vi "SmartSEM Remote API FIB VI slope.vi"(8 "error in":errorcluster, 11 "ActiveX Container":refnum<k7>(container)) -> (0 "error out":errorcluster, 2 "V/I slope":sgl format="%.1g", 3 "reference out":refnum<k7>)   [LabVIEW 2018]
panel:
  in  "Cancel":bool
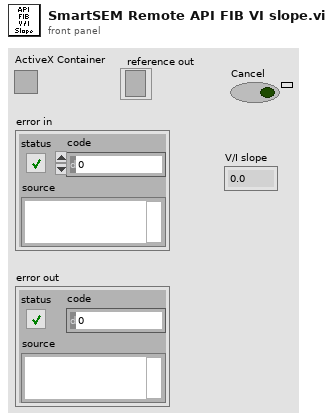
[diagram p1: front panel]
types:
  T1 = cluster{"Filament (A)":sgl, "Accelerator Target (V)":sgl, "Accelerator Actual (V)":sgl, "Extrator Target (V)":sgl, "Extrator Actual (V)":sgl, "Emission Target (uA)":sgl, "Emission Actual (uA)":sgl, "Suppressor (V)":sgl, "Faraday I (nA)":sgl, "Lens1 Target (V)":sgl, "Lens1 Actual (V)":sgl, "Lens2 Target (V)":sgl, "Lens2 Actual (V)":sgl, "Gun Vac (Torr)":sgl, "Column Vac (Torr)":sgl, "Tip Lifetime (uAhr)":sgl}
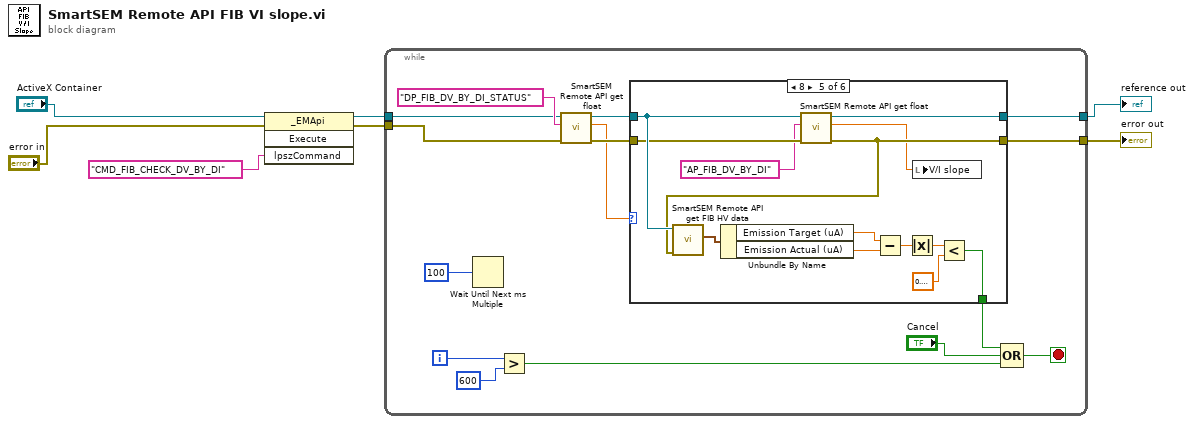
[diagram p0: block diagram]
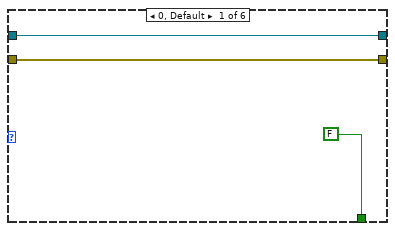
[diagram p2: hidden frame]
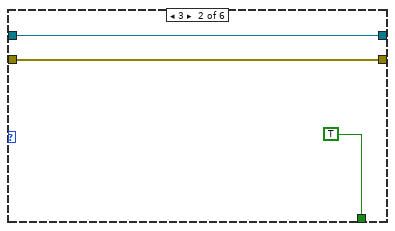
[diagram p3: hidden frame]
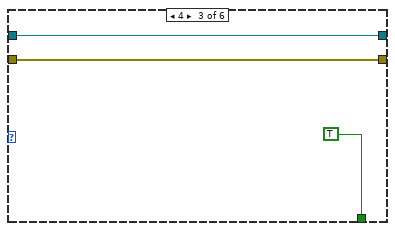
[diagram p4: hidden frame]
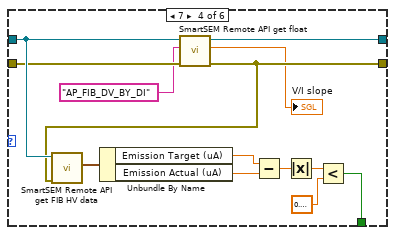
[diagram p5: hidden frame]
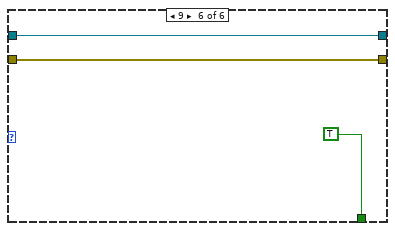
[diagram p6: hidden frame]
diagram:
  n1 = invoke class="_EMApi" method="Execute"(reference="ActiveX Container", error in="error in", "lpszCommand"="CMD_FIB_CHECK_DV_BY_DI") -> (reference out=w6:refnum<k7>, error out=w5:errorcluster)  [unwired: 1 in, 2 out]
  n2 = while {
    tunnel: w6 -> [w10]
    tunnel: w5 -> [w11]
    tunnel: [w22] -> w4
    tunnel: [w21] -> w3
    i -> [w16]
    stop <- w17 stop-if-true
    n3 = Wait Until Next ms Multiple(millisecond multiple=u32 100) -> ()  [unwired: 1 out]
    n4 = Greater?(x=w16, y=600) -> (0:w14:bool)
    n5 = call "SmartSEM Remote API get float.vi"("error in"=w11, "lpszParam"="DP_FIB_DV_BY_DI_STATUS" ("lpszCommand"), "ActiveX Container"=w10) -> ("error out"=w12:errorcluster, "vValue"=w8:sgl, "reference out"=w9:refnum<k7>)  [unwired: 6 in]
    n6 = case shown="8" w8 {
      tunnel: [FALSE TRUE TRUE w41 w54 TRUE] -> w18
      tunnel: w9 -> [w24 w28 w31 w37 w50 w60]
      tunnel: [w24 w28 w31 w34 w47 w60] -> w22
      tunnel: w12 -> [w23 w27 w30 w36 w49 w59]
      tunnel: [w23 w27 w30 w35 w48 w59] -> w21
      frame 0, Default {
      }
      frame 3 {
      }
      frame 4 {
      }
      frame 7 {
        n7 = call "SmartSEM Remote API get float.vi"("error in"=w36, "lpszParam"="AP_FIB_DV_BY_DI" ("lpszCommand"), "ActiveX Container"=w37) -> ("error out"=w35:errorcluster, "vValue"=→"V/I slope":sgl, "reference out"=w34:refnum<k7>)  [unwired: 6 in]
        n8 = call "SmartSEM Remote API get FIB HV data.vi"("error in"=w35, "ActiveX Container"=w37) -> ("Capella HV Data Output"=w38:T1)  [unwired: 6 in, 3 out]
        n9 = Unbundle By Name(w38) -> ("Emission Target (uA)"=w40:sgl, "Emission Actual (uA)"=w39:sgl)
        n10 = Subtract(x=w40, y=w39) -> (x-y=w44:sgl)
        n11 = Absolute Value(x=w44) -> (abs(x)=w43:sgl)
        n12 = Less?(x=w43, y=sgl 0.1) -> (x < y?=w41:bool)
      }
      frame 8 {
        n13 = call "SmartSEM Remote API get float.vi"("error in"=w49, "lpszParam"="AP_FIB_DV_BY_DI" ("lpszCommand"), "ActiveX Container"=w50) -> ("error out"=w48:errorcluster, "vValue"=w45:sgl, "reference out"=w47:refnum<k7>)  [unwired: 6 in]
        n14 = call "SmartSEM Remote API get FIB HV data.vi"("error in"=w48, "ActiveX Container"=w50) -> ("Capella HV Data Output"=w51:T1)  [unwired: 6 in, 3 out]
        n15 = Unbundle By Name(w51) -> ("Emission Target (uA)"=w53:sgl, "Emission Actual (uA)"=w52:sgl)
        n16 = Subtract(x=w53, y=w52) -> (x-y=w57:sgl)
        n17 = Absolute Value(x=w57) -> (abs(x)=w56:sgl)
        n18 = local write "V/I slope"(w45) -> ()
        n19 = Less?(x=w56, y=sgl 0.1) -> (x < y?=w54:bool)
      }
      frame 9 {
      }
    }
    n20 = Compound Arithmetic op=OR(w18, "Cancel", w14) -> (w17:bool)
  }
  "error out" <- w3
  "reference out" <- w4
